vi "Internal DMM.vi"(8 "error in (no error)":errorcluster, 9 "On/Off (T:On)":bool=TRUE, 10 "Check/Set (F:Set)":bool, 11 "VISA Resource Name":refnum<visa-resource-name>) -> (0 "error out":errorcluster, 2 "DMM Enabled":bool, 3 "VISA Resource Name Out":refnum<visa-resource-name>)   [LabVIEW 2012, in "Agilent 34970.lvlib"]
doc: "This VI lets you set/check the state of the internal DMM."
uses:
  <instrlib>/Agilent 34970/Agilent 34970.lvlib
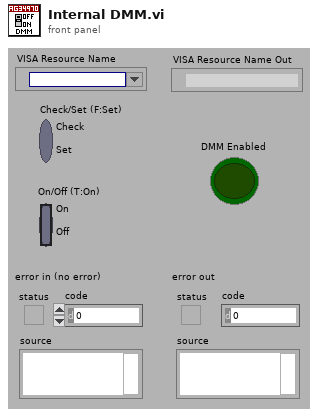
[diagram p1: front panel]
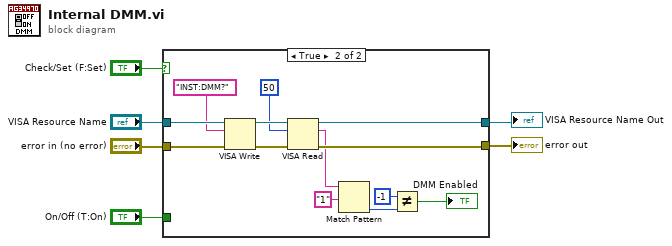
[diagram p0: block diagram]
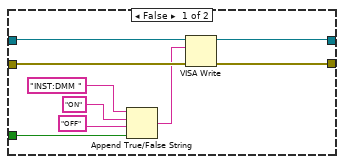
[diagram p2: hidden frame]
diagram:
  n1 = case shown="True" "Check/Set (F:Set)" {
    tunnel: "VISA Resource Name" -> [w13 w28]
    tunnel: "error in (no error)" -> [w12 w27]
    tunnel: [w15 w23] -> w3
    tunnel: [w14 w24] -> w2
    tunnel: "On/Off (T:On)" -> [w7 _]
    frame False {
      n2 = Append True/False String(1:w7, 2:"OFF" ("false string"), 3:"ON" ("true string"), 4:"INST:DMM " ("string (\"\")")) -> (0:w8:string)
      n3 = VISA Write(VISA resource name=w13, write buffer=w8, error in (no error)=w12) -> (VISA resource name out=w15:refnum<visa-resource-name>, error out=w14:errorcluster)  [unwired: 1 out]
    }
    frame True {
      n4 = VISA Write(VISA resource name=w28, write buffer="INST:DMM?", error in (no error)=w27) -> (VISA resource name out=w26:refnum<visa-resource-name>, error out=w25:errorcluster)  [unwired: 1 out]
      n5 = VISA Read(VISA resource name=w26, byte count=u32 50, error in (no error)=w25) -> (VISA resource name out=w23:refnum<visa-resource-name>, read buffer=w17:string, error out=w24:errorcluster)  [unwired: 1 out]
      n6 = Match Pattern(string=w17, regular expression="1") -> (offset past match=w19:i32)  [unwired: 1 in, 3 out]
      n7 = Not Equal?(x=-1, y=w19) -> (x != y?=→"DMM Enabled":bool)
    }
  }
  "error out" <- w2
  "VISA Resource Name Out" <- w3
